vi "Zero Dart.vi"(8 "error in (no error)":errorcluster) -> (0 "error out":errorcluster, 3 "CAN Talon SRX Ref":T1={"DeviceStatus"={"status"=FALSE, "code"=0, "source"=""}, "Type"=enum."PWM", "PWM"={"PWM Channel"=enum."PWM 1", "DeadBand"={"Name"="", "maxPositivePwm"=0, "minPositivePwm"=0, "centerPwm"=0, "maxNegativePwm"=0, "minNegativePwm"=0, "angularRange"=0}}, "CAN"={"Device Number"=0, "Control Mode"=enum."Percent VBus", "Semaphore"=refnum, "Max Vout"=12.0, "TalonSRX Control Mode"=enum."Percent VBus"}, "Invert"=FALSE})   [LabVIEW 2015]
uses:
  <vilib>/Rock Robotics/WPI/MotorControl/WPI_MotorControlDeviceRef.ctl
  <vilib>/Rock Robotics/WPI/MotorControl/WPI_MotorControlType.ctl
  <vilib>/Rock Robotics/SystemInterfaces/DIO/FPGA_DIOPWMChannel.ctl
  <vilib>/Rock Robotics/WPI/PWM/WPI_PWMDeadband.ctl
  <vilib>/Rock Robotics/WPI/CAN/Jaguar/SubVIs/WPI_CANJaguar_ControlMode.ctl
  <vilib>/Rock Robotics/WPI/CAN/TalonSRX/WPI_CANTalonSRX_APIControlMode.ctl
  Robot Global Data.vi
panel:
  out "Offset":dbl
  out "Multiplier":dbl
  out "BottomCount":dbl
  out "TopCount":dbl
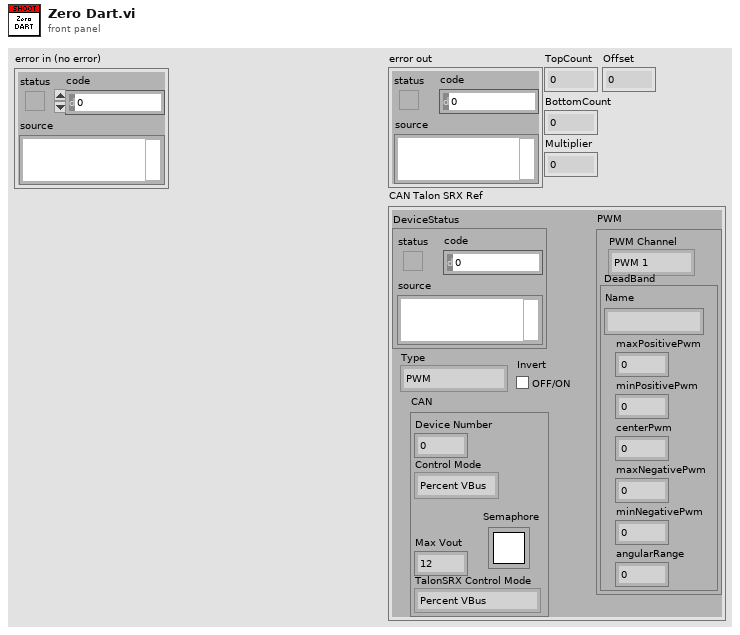
[diagram p1: front panel]
types:
  T1 = typedef "WPI_MotorControlDeviceRef.ctl" = cluster{"DeviceStatus":errorcluster, "Type":T2, "PWM":cluster{"PWM Channel":T3, "DeadBand":T4}, "CAN":cluster{"Device Number":u8, "Control Mode":T5, "Semaphore":T6, "Max Vout":dbl, "TalonSRX Control Mode":T7}, "Invert":bool}
  T2 = typedef "WPI_MotorControlType.ctl" = enum16{"PWM", "CAN", "CANTalonSRX"}
  T3 = typedef "FPGA_DIOPWMChannel.ctl" = enum8{"PWM 0", "PWM 1", "PWM 2", "PWM 3", "PWM 4", "PWM 5", "PWM 6", "PWM 7", "PWM 8", "PWM 9", "PWM MXP 0", "PWM MXP 1", "PWM MXP 2", "PWM MXP 3", "PWM MXP 4", "PWM MXP 5", "PWM MXP 6", "PWM MXP 7", "PWM MXP 8", "PWM MXP 9", "Invalid"}
  T4 = typedef "WPI_PWMDeadband.ctl" = cluster{"Name":string, "maxPositivePwm":i32, "minPositivePwm":i32, "centerPwm":i32, "maxNegativePwm":i32, "minNegativePwm":i32, "angularRange":u16}
  T5 = typedef "WPI_CANJaguar_ControlMode.ctl" = enum8{"Percent VBus", "Current", "Speed", "Position", "Voltage"}
  T6 = typedef "Semaphore RefNum" = refnum<k1>
  T7 = typedef "WPI_CANTalonSRX_APIControlMode.ctl" = enum8{"Percent VBus", "Speed", "Position", "Slave", "Unchanged / Invalid", "Voltage Compensation", "Current", "Motion Profile"}
  T8 = cluster{"Angle Offset":dbl, "Angle Multiplier":dbl, "Max":dbl, "Min":dbl}
  T9 = cluster{"Firing Angle":dbl, "Max Angle?":bool, "Min Angle?":bool}
  T10 = typedef "WPI_DigitalInputDevRef.ctl" = cluster{"DevStatus":errorcluster, "DIO Channel":T11}
  T11 = typedef "FPGA_DIOChannel.ctl" = enum8{"DIO 0", "DIO 1", "DIO 2", "DIO 3", "DIO 4", "DIO 5", "DIO 6", "DIO 7", "DIO 8", "DIO 9", "DIO MXP 0", "DIO MXP 1", "DIO MXP 2", "DIO MXP 3", "DIO MXP 4", "DIO MXP 5", "DIO MXP 6", "DIO MXP 7", "DIO MXP 8", "DIO MXP 9", "DIO MXP 10", "DIO MXP 11", "DIO MXP 12", "DIO MXP 13", "DIO MXP 14", "DIO MXP 15", "Invalid"}
  T12 = typedef "WPI_CANTalonSRX_GlobalStatus.ctl" = cluster{"Applied Throttle":dbl, "Module Enabled":bool, "CAN Error":errorcluster, "Closed Loop Error":dbl, "Forward Limit Switch Closed":bool, "Reverse Limit Switch Closed":bool, "Sensor Position":dbl, "Sensor Velocity":dbl, "Current":dbl, "Sticky Fault - Over Temp":bool, "Sticky Fault - Under Voltage":bool, "Sticky Fault - Forward Limit":bool, "Sticky Fault - Reverse Limit":bool, "Sticky Fault - Forward Soft Limit":bool, "Sticky Fault - Reverse Soft Limit":bool, "Brake is Enabled":bool, "Encoder Position":dbl, "Encoder Velocity":dbl, "Encoder Index Count":dbl, "Encoder A Pin State":bool, "Encoder B Pin State":bool, "Encoder Index Pin State":bool, "Analog In":dbl, "Analog In Velocity":dbl, "Temperature (C)":dbl, "Battery Voltage":dbl, "Control 5 Is Supported":bool, "Current Profile Slot Select":dbl, "Pos Div 8":bool, "Vel Div 4":bool, "Pulse Width Position":i32, "Pulse Width Velocity":i32, "Pulse Width Rise To Rise (us)":i32, "Pulse Width Rise To Fall (us)":i32, "Mot Prof Active Is Under Run":bool, "Mot Prof Active Has Under Run":bool, "Mot Prof Active Is Last":bool, "Mot Prof Active Velocity Only":bool, "Mot Prof Active Is Valid":bool, "Mot Prof Buffer Is Full":bool, "Mot Prof Active Profile Slot Select":i32, "Mot Prof NextID":i32, "Mot Prof Count":i32, "Mot Prof Active Velocity":dbl, "Mot Prof Active Position":dbl, "Mot Prof Output Enable":i32}
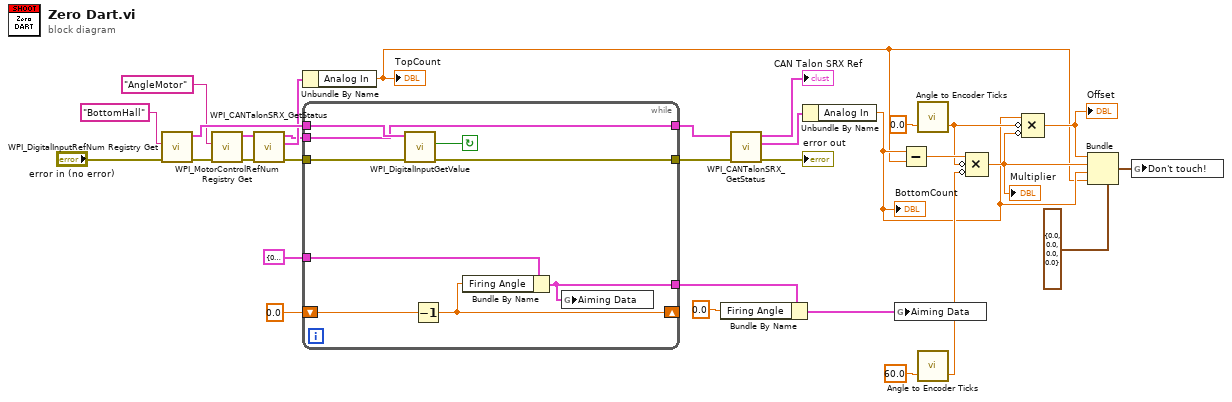
[diagram p0: block diagram]
diagram:
  n1 = call <vilib>:"WPI_DigitalInputRefNum Registry Get.vi"("error in (no error)"="error in (no error)", "refnum name"="BottomHall") -> ("error out"=w19:errorcluster, "DigitalInputDevRef"=w30:T10)  [unwired: 8 in]
  n2 = call <vilib>:"WPI_MotorControlRefNum Registry Get.vi"("error in (no error)"=w19, "refnum name"="AngleMotor") -> ("error out"=w1:errorcluster, "MotorControlDevRef"=w2:T1)  [unwired: 8 in]
  n3 = call <vilib>:"WPI_CANTalonSRX_GetStatus.vi"("error in (no error)"=w1, "CAN Talon SRX Ref"=w2) -> ("error out"=w17:errorcluster, "Talon SRX Status"=w29:T12, "CAN Talon SRX Ref"=w18:T1)  [unwired: 7 in]
  n4 = Unbundle By Name(w29) -> ("Analog In"=w9:dbl)
  "TopCount" <- w9
  n5 = while {
    tunnel: w30 -> [w39]
    tunnel: [w38] -> w16
    tunnel: w18 -> [w38]
    tunnel: w17 -> [w37]
    tunnel: [w36] -> w15
    tunnel: T9 {"Firing Angle"=0.0, "Max Angle?"=FALSE, "Min Angle?"=FALSE} ("Aiming Data") -> [w35]
    tunnel: [w34] -> w4
    shift-right: [w32] -> _
    shift-left: 0.0 -> [w33]
    stop <- w40 continue-if-true
    n6 = call <vilib>:"WPI_DigitalInputGetValue.vi"("error in (no error)"=w37, "DigitalInputDevRef"=w39) -> ("error out"=w36:errorcluster, "Value"=w40:bool)  [unwired: 7 in, 1 out]
    n7 = Decrement(x=w33) -> (x-1=w32:dbl)
    n8 = Bundle By Name(cluster=w35, "Firing Angle"=w32) -> (w34:T9)
    n9 = global write "Robot Global Data.vi" "Aiming Data"(w34) -> ()
  }
  n10 = Bundle By Name(cluster=w4, "Firing Angle"=0.0 ("Output")) -> (w7:T9)
  n11 = call <vilib>:"WPI_CANTalonSRX_GetStatus.vi"("error in (no error)"=w15, "CAN Talon SRX Ref"=w16) -> ("error out"=→"error out":errorcluster, "Talon SRX Status"=w28:T12, "CAN Talon SRX Ref"=→"CAN Talon SRX Ref":T1)  [unwired: 7 in]
  n12 = Unbundle By Name(w28) -> ("Analog In"=w10:dbl)
  "BottomCount" <- w10
  n13 = global write "Robot Global Data.vi" "Aiming Data"(w7) -> ()
  n14 = Subtract(x=w10, y=w9) -> (x-y=w25:dbl)
  n15 = call "Angle to Encoder Ticks.vi"("Angle(degrees)"=0.0) -> ("Dart Length(in)"=w21:dbl)  [unwired: 1 in, 1 out]
  n16 = call "Angle to Encoder Ticks.vi"("Angle(degrees)"=60.0) -> ("Dart Length(in)"=w22:dbl)  [unwired: 1 in, 1 out]
  n17 = Compound Arithmetic op=MULTIPLY(w25, invert w21, invert w22) -> (w11:dbl)
  "Multiplier" <- w11
  n18 = Compound Arithmetic op=MULTIPLY(w10, invert w21, invert w11) -> (w12:dbl)
  "Offset" <- w12
  n19 = Bundle(cluster=T8 {"Angle Offset"=0.0, "Angle Multiplier"=0.0, "Max"=0.0, "Min"=0.0} ("Don't touch!"), "Angle Offset"=w12, "Angle Multiplier"=w11, "Max"=w10, "Min"=w9) -> (w13:T8)
  n20 = global write "Robot Global Data.vi" "Don't touch!"(w13) -> ()
